vi "Get Head Temperature.vi"(0 "Device ID (0)":i32, 11 "error in (no error)":errorcluster {"code" format="%.0x"}) -> (4 "Device ID out":i32, 6 "Sensor Temperature":i16, 8 "Processor Temperature":i16, 10 "Case Temperature":i16, 15 "error out":errorcluster {"code" format="%.0x"})   [LabVIEW 2020, in "KEYENCE LJ-X8000A.lvlib"]
doc: "This function reads the head temperature.\nTemperature format: Signed. When the value is xxxxx (decimal), the temperature is\nexpressed in Celsius as xxx.xx degrees.\n<B>Note</B>:\nThe temperature of the processor and case cannot be acquired with the LJ-V head.\n(0xFFFF is returned.)"
uses:
  KEYENCE LJ-X8000A.lvlib
panel:
  # "(c) 2019 KEYENCE CORPORATION.  ALL RIGHTS RESERVED."
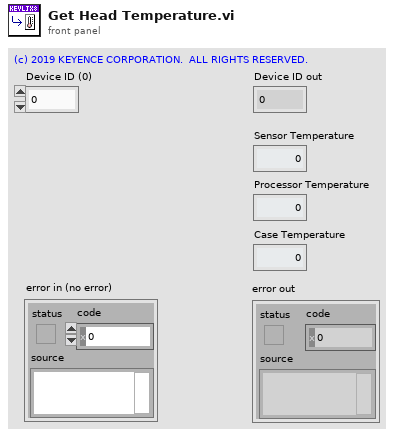
[diagram p1: front panel]
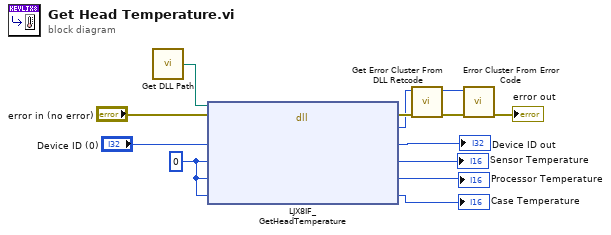
[diagram p0: block diagram]
diagram:
  w6 = i16 0 ("pnSensorTemperature")
  n1 = call "Get DLL Path.vi"() -> ("DLL Path"=w10:path)  [unwired: 3 in]
  n2 = dll-call lib="C:/Program Files (x86)/National Instruments/LabVIEW 2018/instr.lib/KEYENCE LJ-X8000/LJX8_IF.*" fn="LJX8IF_GetHeadTemperature"(path in=w10, error in="error in (no error)", "lDeviceId"="Device ID (0)", "pnSensorTemperature"=w6, "pnProcessorTemperature"=w6, "pnCaseTemperature"=w6) -> (error out=w8:errorcluster, "lRetCode"=w7:i32, "lDeviceId"=→"Device ID out":i32, "pnSensorTemperature"=→"Sensor Temperature":i16, "pnProcessorTemperature"=→"Processor Temperature":i16, "pnCaseTemperature"=→"Case Temperature":i16)  [unwired: 1 in, 1 out]
  n3 = call "Get Error Cluster From DLL Retcode.vi"("error in (no error)"=w8, "DLL Return Code"=w7) -> ("error out"=w9:errorcluster, "VI Error Code"=w1:i32)  [unwired: 8 in]
  n4 = call <vilib>:"Error Cluster From Error Code.vi"("error in (no error)"=w9, "error code (0)"=w1) -> ("error out"=→"error out":errorcluster)  [unwired: 7 in]
